vi "RemoveShape Response.vi"(8 "error in (no error)":errorcluster, 10 "Indexes":i32[](array[numeric]), 11 "Image Editor Handler in":refnum<class "Image Editor Handler.lvclass">) -> (0 "error out":errorcluster, 3 "Image Editor Handler out":refnum<class "Image Editor Handler.lvclass">)   [LabVIEW 2015, in "LV Image Editor Framework.lvlib" / "Image Editor Handler.lvclass"]
uses:
  Image Editor Handler.lvclass
  Image Editor Handler.lvclass/Image Editor Handler.ctl
  Image/Image.lvclass
  Forms/Shape/Shape.lvclass
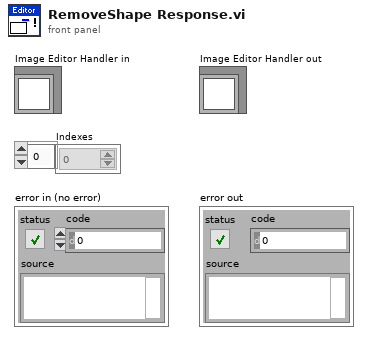
[diagram p1: front panel]
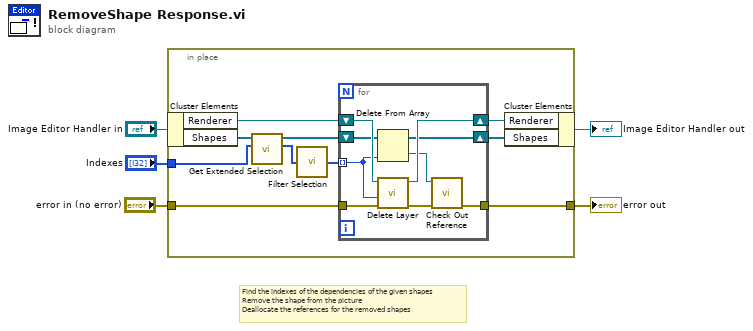
[diagram p0: block diagram]
diagram:
  # "Find the indexes of the dependencies of the given shapes\nRemove the shape from the picture\nDeallocate the references for the removed shapes"
  n1 = in-place {
    in-place-border: "error in (no error)" -> [w13]
    in-place-border: [w11] -> w4
    in-place-border: "Indexes" -> [w7]
    n2 = in-place-cluster #1("Image Editor Handler in") -> ("Renderer"=w15:refnum<class "Image.lvclass">, "Shapes"=w10:refnum<data-value>[])
    n3 = call "Get Extended Selection.vi"("Selected"=w7, "Shapes"=w10) -> ("Ext. Selection"=w8:i32[], "Shapes out"=w9:refnum<data-value>[])  [unwired: 7 in, 1 out]
    n4 = call "Filter Selection.vi"("Ext. Selection"=w8) -> ("Filtered Selection"=w6:i32[])  [unwired: 4 in]
    n5 = for {
      shift-right: [w23] -> w14
      shift-left: w15 -> [w24]
      tunnel: w6 -> [w19] mode=indexing
      tunnel: w13 -> [w22]
      shift-right: [w20] -> w12
      shift-left: w9 -> [w21]
      tunnel: [w16] -> w11
      n6 = Delete From Array(array=w21, index=w19) -> (deleted portion=w18:refnum<data-value>, array with subset deleted=w20:refnum<data-value>[])  [unwired: 1 in]
      n7 = call "Delete Layer.vi"("error in (no error)"=w22, "Layer Index"=w19, "Image in"=w24) -> ("error out"=w17:errorcluster, "Image out"=w23:refnum<class "Image.lvclass">)  [unwired: 7 in]
      n8 = call "Check Out Reference.vi"("error in (no error)"=w17, "Shape Reference"=w18) -> ("error out"=w16:errorcluster)  [unwired: 9 in]
    }
    n9 = in-place-cluster #1("Renderer"=w14, "Shapes"=w12) -> (→"Image Editor Handler out":refnum<class "Image Editor Handler.lvclass">)
  }
  "error out" <- w4
